vi "keyboardAcquire_pR.vi"(0 "device ID":refnum<k1>, 5 "error in (no error)":errorcluster) -> (14 "device ID":refnum<k1>, 15 "key pressed":T1(ring), 19 "error out":errorcluster)   [LabVIEW 2014]
doc: "Returns data about the device connected to the computer. Wire data to the <B>device ID</B> input to determine the polymorphic instance to use or manually select the instance."
uses:
  <resource>/lvinput.dll
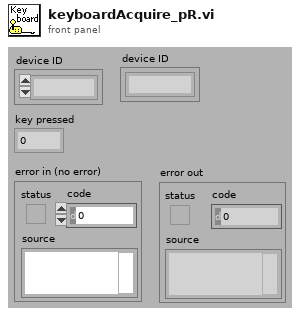
[diagram p1: front panel]
types:
  T1 = enum16{"0", "1", "2", "3", "4", "5", "6", "7", "8", "9", "A", "B", "C", "D", "E", "F", "G", "H", "I", "J", "K", "L", "M", "N", "O", "P", "Q", "R", "S", "T", "U", "V", "W", "X", "Y", "Z", "F1", "F2", "F3", "F4", "F5", "F6", "F7", "F8", "F9", "F10", "F11", "F12", "F13", "F14", "F15", "ADD", "BACK", "BACKSLASH", "CAPITAL", "COMMA", "DECIMAL", "DELETE", "DIVIDE", "DOWN", "END", "EQUALS", "ESCAPE", "GRAVE (`)", "HOME", "INSERT", "LBRACKET", "LCONTROL", "LEFT", "L ALT", "LSHIFT", "LWIN", "MINUS", "MULTIPLY", "NEXT", "NUMLOCK", "NUMPAD_0", "NUMPAD_1", "NUMPAD_2", "NUMPAD_3", "NUMPAD_4", "NUMPAD_5", "NUMPAD_6", "NUMPAD_7", "NUMPAD_8", "NUMPAD_9", "PAUSE", "PERIOD", "PRIOR (PG UP)", "RBRACKET", "RCONTROL", "RETURN", "RIGHT", "R ALT", "RSHIFT", "RWIN", "SCROLL", "SEMICOLON", "SLASH", "SPACE", "SUBTRACT", "TAB", "UP", "ENTER (num pad)", "' (quote)"}
  T2 = enum16{"0", "1", "2", "3", "4", "5", "6", "7", "8", "9", "A", "B", "C", "D", "E", "F", "G", "H", "I", "J", "K", "L", "M", "N", "O", "P", "Q", "R", "S", "T", "U", "V", "W", "X", "Y", "Z", "F1", "F2", "F3", "F4", "F5", "F6", "F7", "F8", "F9", "F10", "F11", "F12", "F13", "F14", "F15", "ADD", "BACK", "BACKSLASH", "CAPITAL", "COMMA", "DECIMAL", "DELETE", "DIVIDE", "DOWN", "END", "EQUALS", "ESCAPE", "GRAVE (`)", "HOME", "INSERT", "LBRACKET", "LCONTROL", "LEFT", "L ALT", "LSHIFT", "LWIN", "MINUS", "MULTIPLY", "NEXT", "NUMLOCK", "NUMPAD_0", "NUMPAD_1", "NUMPAD_2", "NUMPAD_3", "NUMPAD_4", "NUMPAD_5", "NUMPAD_6", "NUMPAD_7", "NUMPAD_8", "NUMPAD_9", "PAUSE", "PERIOD", "PRIOR (PG UP)", "RBRACKET", "RCONTROL", "RETURN", "RIGHT", "R ALT", "RSHIFT", "RWIN", "SCROLL", "SEMICOLON", "SLASH", "SPACE", "SUBTRACT", "TAB", "UP", "ENTER (num pad)", "' (quote)"}[]
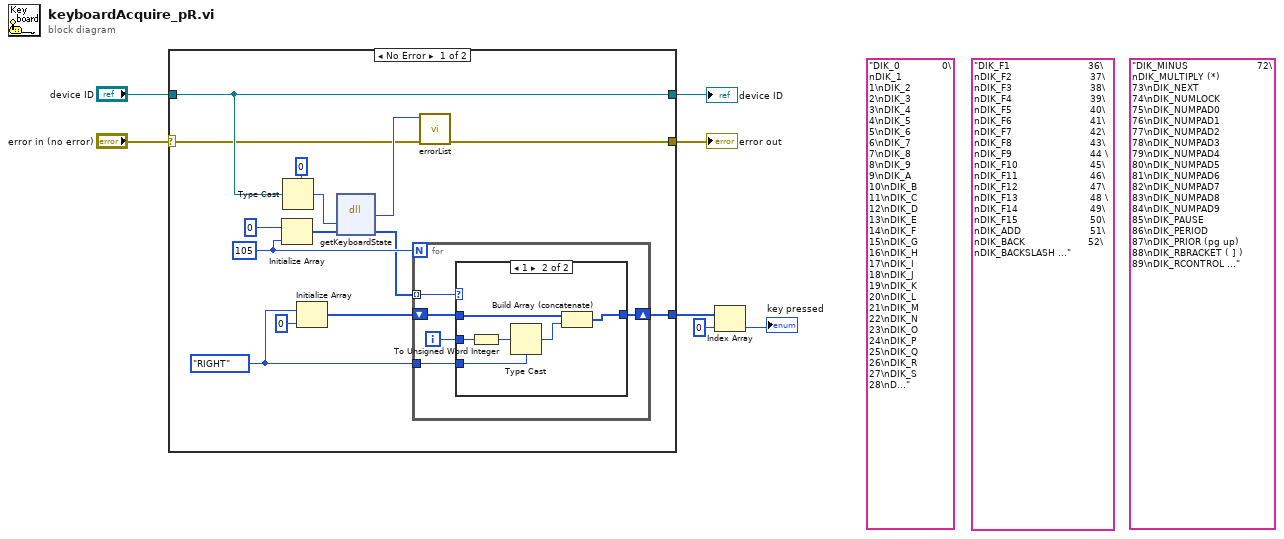
[diagram p0: block diagram]
diagram:
  (unwired) "DIK_MINUS                       72\nDIK_MULTIPLY (*)             73\nDIK_NEXT                          74\nDIK_NUMLOCK                  75\nDIK_NUMPAD0                  76\nDIK_NUMPAD1                  77\nDIK_NUMPAD2                  78\nDIK_NUMPAD3                  79\nDIK_NUMPAD4                  80\nDIK_NUMPAD5                  81\nDIK_NUMPAD6                  82\nDIK_NUMPAD7                  83\nDIK_NUMPAD8                  84\nDIK_NUMPAD9                  85\nDIK_PAUSE                       86\nDIK_PERIOD                     87\nDIK_PRIOR (pg up)           88\nDIK_RBRACKET ( ] )          89\nDIK_RCONTROL               90\nDIK_RETURN                    91\nDIK_RIGHT                       92\nDIK_RMENU (R ALT)         93\nDIK_RSHIFT (R shift)       94\nDIK_RWIN (R win)            95\nDIK_SCROLL                     96\nDIK_SEMICOLON              97\nDIK_SLASH                       98\nDIK_SPACE                       99\nDIK_SUBTRACT               100\nDIK_TAB                          101\nDIK_UP                            102\nDIR_ENTER(NUM)           103\nDIR_APOSTROPHY         104"
  (unwired) "DIK_F1                          36\nDIK_F2                          37\nDIK_F3                          38\nDIK_F4                          39\nDIK_F5                          40\nDIK_F6                          41\nDIK_F7                          42\nDIK_F8                          43\nDIK_F9                          44 \nDIK_F10                        45\nDIK_F11                        46\nDIK_F12                        47\nDIK_F13                        48 \nDIK_F14                        49\nDIK_F15                        50\nDIK_ADD                       51\nDIK_BACK                     52\nDIK_BACKSLASH           53\nDIK_CAPITAL                54\nDIK_COMMA                 55\nDIK_DECIMAL               56\nDIK_DELETE                  57\nDIK_DIVIDE                  58\nDIK_DOWN                   59\nDIK_END                       60\nDIK_EQUALS                 61\nDIK_ESCAPE                 62\nDIK_GRAVE (`)             63\nDIK_HOME                    64\nDIK_INSERT                  65\nDIK_LBRACKET             66\nDIK_LCONTROL            67\nDIK_LEFT                      68\nDIK_LMENU (L ALT)      69\nDIK_LSHIFT                  70\nDIK_LWIN                    71\n\n\n\n\n\n\n"
  (unwired) "DIK_0              0\nDIK_1              1\nDIK_2              2\nDIK_3              3\nDIK_4              4\nDIK_5              5\nDIK_6              6\nDIK_7              7\nDIK_8              8\nDIK_9              9\nDIK_A            10\nDIK_B             11\nDIK_C            12\nDIK_D            13\nDIK_E             14\nDIK_F             15\nDIK_G            16\nDIK_H            17\nDIK_I             18\nDIK_J             19\nDIK_K             20\nDIK_L             21\nDIK_M            22\nDIK_N            23\nDIK_O            24\nDIK_P             25\nDIK_Q            26\nDIK_R            27\nDIK_S             28\nDIK_T             29\nDIK_U            30\nDIK_V             31\nDIK_W           32\nDIK_X             33\nDIK_Y             34\nDIK_Z             35\n\n"
  n1 = case shown="No Error" "error in (no error)" {
    selector: "error in (no error)" -> [w13 w34]
    tunnel: [w14 w34] -> w7
    tunnel: "device ID" -> [w15 w35]
    tunnel: [w15 w35] -> w5
    tunnel: [w8 _] -> w1
    frame No Error {
      w10 = T1."RIGHT" ("key type")
      w19 = 105 ("Dimension Size")
      n2 = Initialize Array(i8 0, w19) -> (w21:i8[])
      n3 = Type Cast(type=0 ("Input Value"), x=w15) -> (*(type *) &x=w16:i32)
      n4 = Initialize Array(w10, 0 ("dimension size")) -> (w11:T2)
      n5 = dll-call lib="C:/Program Files (x86)/National Instruments/LabVIEW 2014/resource/lvinput.*" fn="getKeyboardState"(w16, w21) -> (w20:i32, w18:i8[])  [unwired: 4 in, 2 out]
      n6 = for {
        N: w19 -> [_]
        tunnel: w18 -> [w26] mode=indexing
        shift-right: [w24] -> w8
        shift-left: w11 -> [w25]
        tunnel: w10 -> [w22]
        i -> [w23]
        n7 = case shown="1" w26 {
          tunnel: w25 -> [w27 w32]
          tunnel: [w27 w33] -> w24
          tunnel: w23 -> [_ w31]
          tunnel: w22 -> [_ w30]
          frame 0, Default {
          }
          frame 1 {
            n8 = To Unsigned Word Integer(number=w31) -> (unsigned 16bit integer=w29:u16)
            n9 = Type Cast(type=w30, x=w29) -> (*(type *) &x=w28:T1)
            n10 = Build Array (concatenate)(w32, w28) -> (w33:T2)
          }
        }
      }
      n11 = call <vilib>:"errorList.vi"("error in (no error)"=w13, "error code"=w20) -> ("error out"=w14:errorcluster)  [unwired: 9 in]
    }
    frame Error {
    }
  }
  "error out" <- w7
  "device ID" <- w5
  n12 = Index Array(array=w1, index=0) -> (element=→"key pressed":T1)
